vi "lo read.vi"(7 "len":u32, 8 "error in (no error)":errorcluster, 9 "buf":string, 10 "fd":i32) -> (0 "error out":errorcluster, 1 "lo_read":i32, 2 "buf out":string)   [LabVIEW 2019, in "libpqlv64.lvlib"]
uses:
  libpqlv64.lvlib
  libpq.dll
panel:
  in  "conn":u32
  out "conn_out":u32
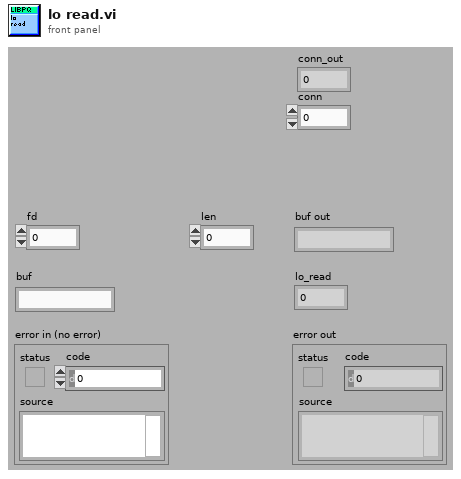
[diagram p1: front panel]
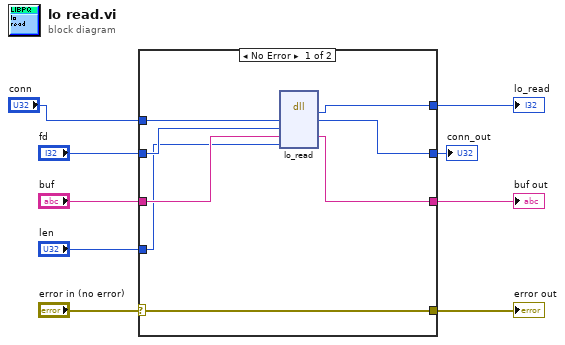
[diagram p0: block diagram]
diagram:
  n1 = case shown="No Error" "error in (no error)" {
    selector: "error in (no error)" -> [w17 w20]
    tunnel: [w17 w20] -> w8
    tunnel: [w16 _] -> w7
    tunnel: [w15 w18] -> w2
    tunnel: "fd" -> [w14 _]
    tunnel: "buf" -> [w13 w19]
    tunnel: [w12 w19] -> w4
    tunnel: "len" -> [w11 _]
    tunnel: "conn" -> [w10 w18]
    frame No Error {
      n2 = dll-call lib="libpq.*" fn="lo_read"("conn"=w10, "fd"=w14, "buf"=w13, "len"=w11) -> ("lo_read"=w16:i32, "conn"=w15:u32, "buf"=w12:string)  [unwired: 5 in, 2 out]
    }
    frame Error {
    }
  }
  "lo_read" <- w7
  "buf out" <- w4
  "error out" <- w8
  "conn_out" <- w2
